vi "Write 4 Bits.vi"(8 "error in (no error)":errorcluster, 9 "Value":u8, 10 "VISA resource name in":refnum<visa-resource-name>, 11 "LCD-I2C in":refnum<class "LCD-I2C.lvclass">) -> (0 "error out":errorcluster, 2 "VISA resource name":refnum<visa-resource-name>, 3 "LCD-I2C out":refnum<class "LCD-I2C.lvclass">)   [LabVIEW 2020, in "CTI-Visa-DeviceLib.lvlib" / "LCD-I2C.lvclass"]
uses:
  LCD-I2C.lvclass
  LCD-I2C.lvclass/LCD-I2C.ctl
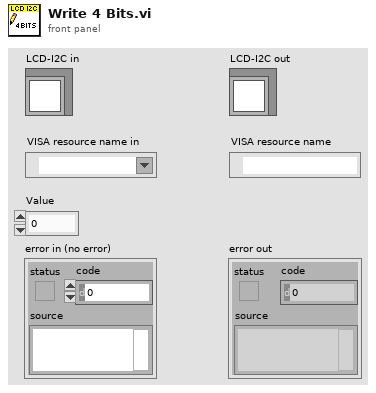
[diagram p1: front panel]
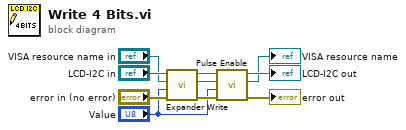
[diagram p0: block diagram]
diagram:
  n1 = call "Expander Write.vi"("error in (no error)"="error in (no error)", "Value"="Value", "VISA resource name in"="VISA resource name in", "LCD-I2C in"="LCD-I2C in") -> ("error out"=w5:errorcluster, "VISA resource name"=w4:refnum<visa-resource-name>, "LCD-I2C out"=w9:refnum<class "LCD-I2C.lvclass">)  [unwired: 5 in]
  n2 = call "Pulse Enable.vi"("error in (no error)"=w5, "Value"="Value", "VISA resource name in"=w4, "LCD-I2C in"=w9) -> ("error out"=→"error out":errorcluster, "VISA resource name"=→"VISA resource name":refnum<visa-resource-name>, "LCD-I2C out"=→"LCD-I2C out":refnum<class "LCD-I2C.lvclass">)  [unwired: 5 in]
